vi "Validate Channel or Section Name.vi"(8 "error in (no error)":errorcluster, 10 "Name In":string, 11 "Refnum In":T1 format="%.0x") -> (0 "error out":errorcluster, 2 "Name Out":string, 3 "Refnum Out":T1 format="%.0x")   [LabVIEW 2018, in "Instrument Addon Scripting API.lvlib"]
uses:
  Instrument Addon Scripting API.lvlib
  <vilib>/NI Veristand/Custom Device API/Custom Device Item Ref.ctl
  <vilib>/Utility/error.llb/Error Cluster From Error Code.vi
  <vilib>/ErrorRing/Error Ring.xnode
  <vilib>/NI Veristand/Custom Device Tools/Custom Device Utility Library/Custom Device Utility Library.lvlib
  <vilib>/NI Veristand/Custom Device API/Custom Device API.lvlib
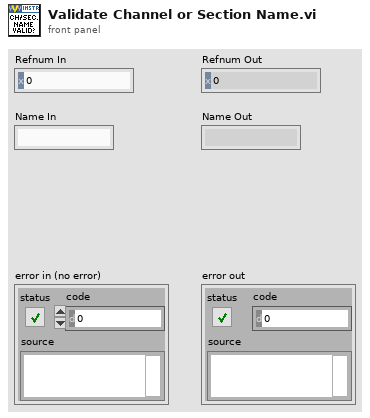
[diagram p1: front panel]
types:
  T1 = typedef "Custom Device API.lvlib/Custom Device Item Ref.ctl" = u64
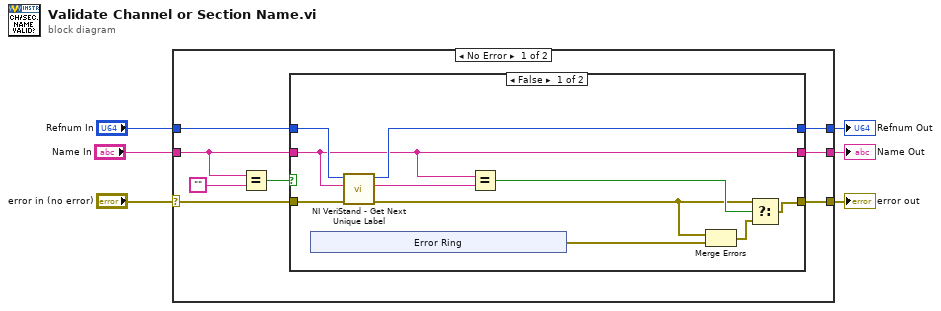
[diagram p0: block diagram]
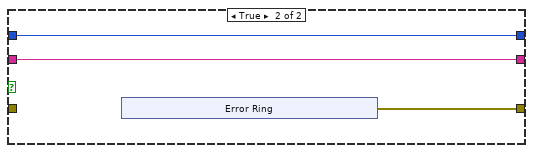
[diagram p2: hidden frame]
diagram:
  n1 = case shown="No Error" "error in (no error)" {
    selector: "error in (no error)" -> [w7 w40]
    tunnel: [w14 w39] -> w6
    tunnel: [w13 w40] -> w5
    tunnel: "Refnum In" -> [w12 w39]
    tunnel: "Name In" -> [w9 w38]
    tunnel: [w8 w38] -> w2
    frame No Error {
      n2 = Equal?(x=w9, y="") -> (x = y?=w10:bool)
      n3 = case shown="False" w10 {
        tunnel: [w24 w32] -> w14
        tunnel: [w18 w30] -> w13
        tunnel: w7 -> [w23 _]
        tunnel: w12 -> [w22 w32]
        tunnel: w9 -> [w20 w31]
        tunnel: [w20 w31] -> w8
        frame False {
          n4 = xnode "Error Ring"() -> ("error out"=w15:errorcluster)
          n5 = call <vilib>:"NI VeriStand - Get Next Unique Label.vi"("error in (no error)"=w23, "Label"=w20, "Parent Ref in"=w22) -> ("error out"=w16:errorcluster, "Label out"=w21:string, "Parent Ref dup"=w24:T1)  [unwired: 5 in, 1 out]
          n6 = Equal?(x=w20, y=w21) -> (x = y?=w19:bool)
          n7 = Merge Errors(w16, w15) -> (w17:errorcluster)
          n8 = Select(t=w16, s=w19, f=w17) -> (s? t:f=w18:errorcluster)
        }
        frame True {
          n9 = xnode "Error Ring"() -> ("error out"=w30:errorcluster)
        }
      }
    }
    frame Error {
    }
  }
  "Refnum Out" <- w6
  "error out" <- w5
  "Name Out" <- w2
